vi "MSEditor_StringCtlEncolour&Font.vi"(8 "error in (no error)":errorcluster, 9 "SELs":cluster{"Start":u32, "End":u32}[](array[cluster]), 10 "TextProperties":T1, 11 "String ctl ref":refnum<vi>) -> (0 "error out":errorcluster, 3 "String ctl ref out":refnum<vi>)   [LabVIEW 2018]
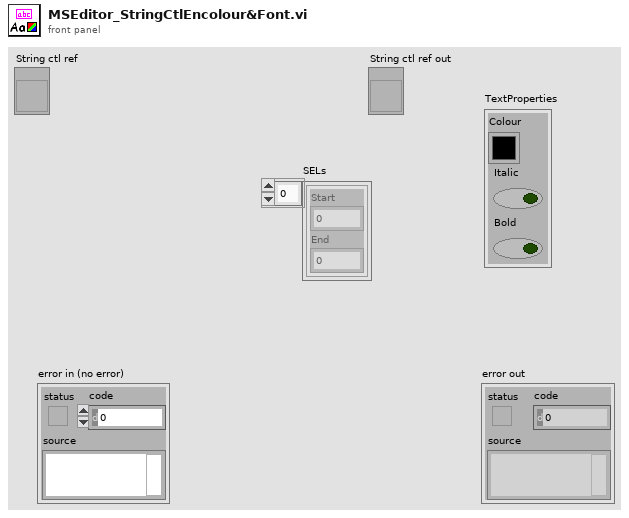
[diagram p1: front panel]
types:
  T1 = cluster{"Colour":u32, "Italic":bool, "Bold":bool}
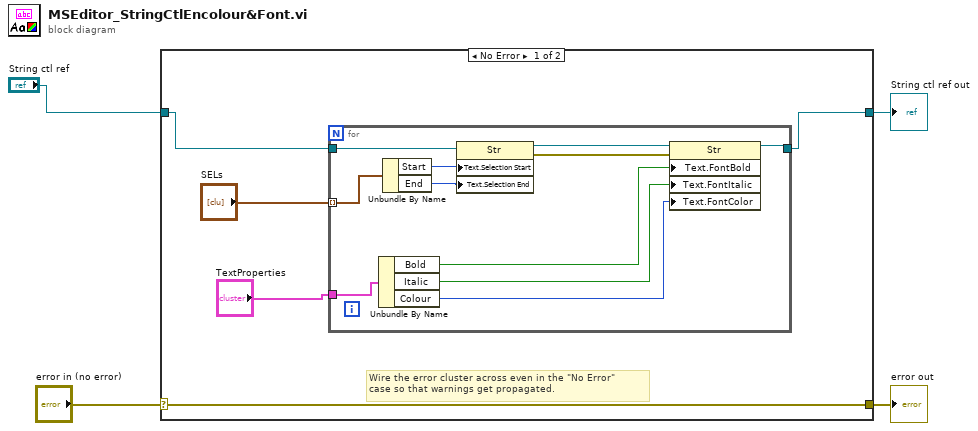
[diagram p0: block diagram]
diagram:
  n1 = case shown="No Error" "error in (no error)" {
    selector: "error in (no error)" -> [w9 w22]
    tunnel: [w9 w22] -> w3
    tunnel: "String ctl ref" -> [w8 w21]
    tunnel: [w7 w21] -> w1
    frame No Error {
      # "Wire the error cluster across even in the \"No Error\"\ncase so that warnings get propagated."
      n2 = for {
        tunnel: "SELs" -> [w18] mode=indexing
        tunnel: "TextProperties" -> [w16]
        tunnel: w8 -> [w17]
        tunnel: [w14] -> w7
        n3 = Unbundle By Name(w16) -> ("Bold"=w13:bool, "Italic"=w12:bool, "Colour"=w10:u32)
        n4 = Unbundle By Name(w18) -> ("Start"=w20:u32, "End"=w19:u32)
        n5 = property class="Str"(reference=w17, "Text.Selection Start"=w20, "Text.Selection End"=w19) -> (reference out=w15:refnum<vi>, error out=w11:errorcluster)  [unwired: 1 in]
        n6 = property class="Str"(reference=w15, error in=w11, "Text.FontBold"=w13, "Text.FontItalic"=w12, "Text.FontColor"=w10) -> (reference out=w14:refnum<vi>)  [unwired: 1 out]
      }
    }
    frame Error {
    }
  }
  "error out" <- w3
  "String ctl ref out" <- w1
